vi "API - Parse Config File.vi"(8 "error in (no error)":errorcluster, 10 "Config Path":path, 11 "Node Ptr":T1 format="%.0x") -> (0 "error out":errorcluster, 1 "Descriptions":string[](array[string]), 2 "Channel Configuration":string[][](array[string]))   [LabVIEW 2016, in "UDP-Custom-Device System Explorer.lvlib"]
uses:
  UDP-Custom-Device System Explorer.lvlib
  <vilib>/NI Veristand/Custom Device API/Custom Device Item Ref.ctl
  <vilib>/Utility/file.llb/Read Delimited Spreadsheet (string).vi
  <vilib>/NI VeriStand/Custom Device API/Custom Device API.lvlib
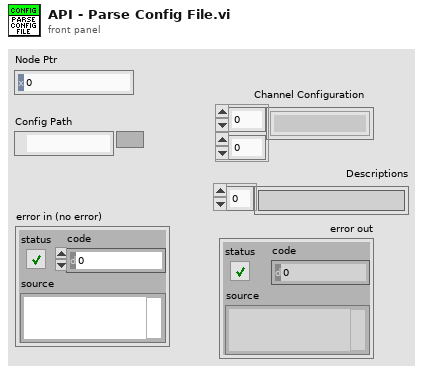
[diagram p1: front panel]
types:
  T1 = typedef "Custom Device API.lvlib/Custom Device Item Ref.ctl" = u64
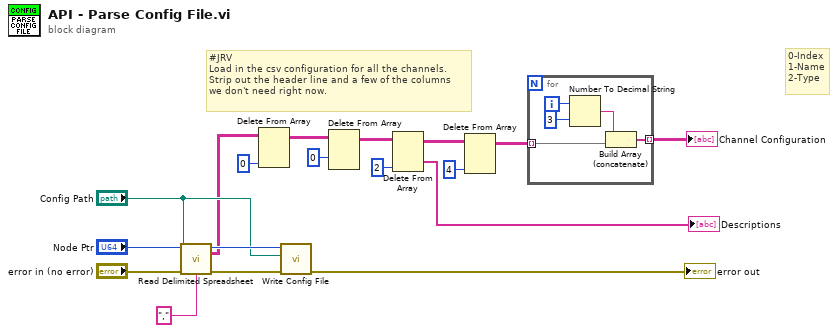
[diagram p0: block diagram]
diagram:
  # "0-Index\n1-Name\n2-Type"
  # "#JRV\nLoad in the csv configuration for all the channels.\nStrip out the header line and a few of the columns\nwe don't need right now."
  n1 = call-poly <vilib>:"Read Delimited Spreadsheet.vi"("file path (dialog if empty)"="Config Path", "error in (no error)"="error in (no error)", "delimiter (\\t)"="," ("delimiter (\\t)")) -> ("all rows"=w11:string[][], "error out"=w13:errorcluster)  [unwired: 7 in, 4 out]
  n2 = Delete From Array(array=w11, index (col)=0 ("index (row)")) -> (array with subset deleted=w7:string[][])  [unwired: 2 in, 1 out]
  n3 = call "Write Config File.vi"("error in (no error)"=w13, "Config File"="Config Path", "Node Ptr"="Node Ptr") -> ("error out"=→"error out":errorcluster)  [unwired: 7 in, 1 out]
  n4 = Delete From Array(array=w7, index (row)=0) -> (array with subset deleted=w6:string[][])  [unwired: 2 in, 1 out]
  n5 = Delete From Array(array=w6, index (col)=2 ("disabled index (col)")) -> (deleted portion=→"Descriptions":string[], array with subset deleted=w3:string[][])  [unwired: 2 in]
  n6 = Delete From Array(array=w3, index (col)=4 ("disabled index (col)")) -> (array with subset deleted=w2:string[][])  [unwired: 2 in, 1 out]
  n7 = for {
    tunnel: w2 -> [w22] mode=indexing
    tunnel: [w18] -> w8 mode=indexing
    i -> [w21]
    n8 = Number To Decimal String(number=w21, width (-)=i16 3) -> (decimal integer string=w19:string)
    n9 = Build Array (concatenate)(w19, w22) -> (w18:string[])
  }
  "Channel Configuration" <- w8
